vi "New Assert Message.vi"(8 "error in (no error)":errorcluster, 10 "Assert Message":string, 11 "Main Display in":refnum<class "Main Display.lvclass">) -> (0 "error out":errorcluster, 3 "Main Display out":refnum<class "Main Display.lvclass">)   [LabVIEW 2016, in "Assert API Components.lvlib" / "Assert Display.lvlib" / "Main Display.lvlib" / "Main Display.lvclass"]
uses:
  Main Display.lvclass
  Assert API Components/Message Data.ctl
  Assert API Components/VI References.ctl
  Main Display.lvclass/Main Display.ctl
  Display Configurations/Base Display Configuration.lvclass
  Assert API Components/Assert API Components.lvlib
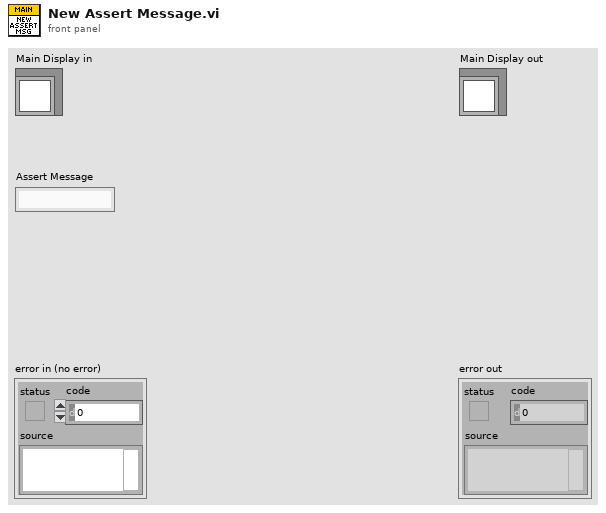
[diagram p1: front panel]
types:
  T1 = typedef "Assert API Components.lvlib/Message Data.ctl" = cluster{"Data Value":variant, "Last Update":timestamp, "Comment":string, "Evaluation String":string, "Status":bool, "Assert Name":string, "Failure Action":string, "Assert VI Name":string, "Calling VI Name":string, "Assert VI UID":i32, "Top Level VI Name":string, "VI References":T2, "Assert Build Timestamp":timestamp, "Assert Builder User Name":string, "Data Type":string}
  T2 = typedef "Assert API Components.lvlib/VI References.ctl" = cluster{"Calling VI Ref":refnum<vi>, "Assert VI Ref":refnum<vi>}
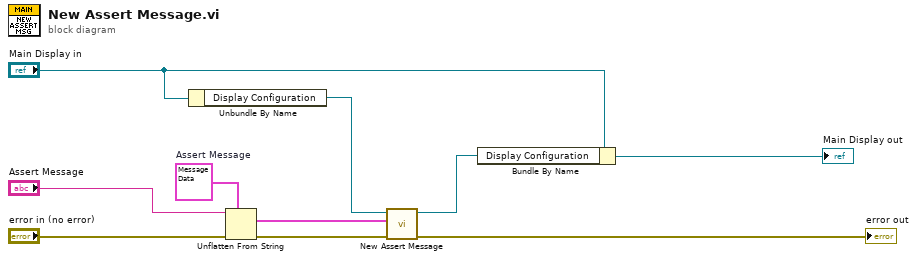
[diagram p0: block diagram]
diagram:
  w7 = T1 {"Data Value"=variant, "Last Update"=timestamp(0 s since 1904-01-01), "Comment"="", "Evaluation String"="", "Status"=FALSE, "Assert Name"="", "Failure Action"="", "Assert VI Name"="", "Calling VI Name"="", "Assert VI UID"=0, "Top Level VI Name"="", "VI References"={"Calling VI Ref"=refnum, "Assert VI Ref"=refnum}, "Assert Build Timestamp"=timestamp(0 s since 1904-01-01), "Assert Builder User Name"="", "Data Type"=""}  # Assert Message
  n1 = Unbundle By Name("Main Display in") -> ("Display Configuration"=w4:refnum<class "Base Display Configuration.lvclass">)
  n2 = Unflatten From String(type=w7, binary string="Assert Message", error in (no error)="error in (no error)") -> (value=w1:T1, error out=w9:errorcluster)  [unwired: 2 in, 1 out]
  n3 = call-dynamic "New Assert Message.vi"("error in (no error)"=w9, "Assert Message"=w1, "Base Display Configuration in"=w4) -> ("error out"=→"error out":errorcluster, "Base Display Configuration out"=w3:refnum<class "Base Display Configuration.lvclass">)  [unwired: 7 in]
  n4 = Bundle By Name(cluster="Main Display in", "Display Configuration"=w3) -> (→"Main Display out":refnum<class "Main Display.lvclass">)
